vi "setBoundaries.vi"(8 "error in (no error)":errorcluster, 10 "Boundaries":T1, 11 "Rectangle in":refnum<class "Rectangle.lvclass">) -> (0 "error out":errorcluster, 3 "Rectangle out":refnum<class "Rectangle.lvclass">)   [LabVIEW 2010, in "Rectangle.lvclass"]
uses:
  Rectangle.lvclass
  Rectangle.lvclass/Rectangle.ctl
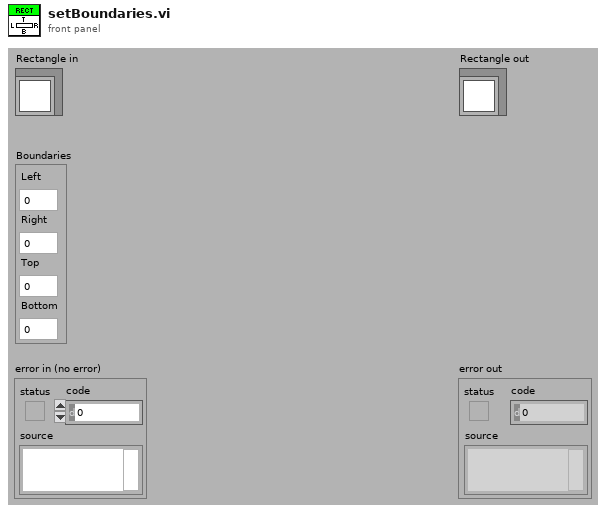
[diagram p1: front panel]
types:
  T1 = cluster{"Left":dbl, "Right":dbl, "Top":dbl, "Bottom":dbl}
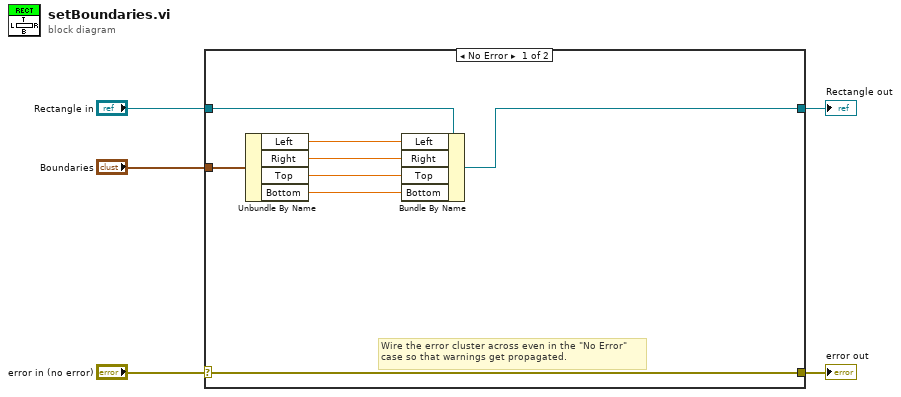
[diagram p0: block diagram]
diagram:
  n1 = case shown="No Error" "error in (no error)" {
    selector: "error in (no error)" -> [w13 w15]
    tunnel: [w13 w15] -> w4
    tunnel: [w11 w14] -> w2
    tunnel: "Rectangle in" -> [w12 w14]
    tunnel: "Boundaries" -> [w10 _]
    frame No Error {
      # "Wire the error cluster across even in the \"No Error\"\ncase so that warnings get propagated."
      n2 = Unbundle By Name(w10) -> ("Left"=w9:dbl, "Right"=w8:dbl, "Top"=w7:dbl, "Bottom"=w6:dbl)
      n3 = Bundle By Name(cluster=w12, "Left"=w9, "Right"=w8, "Top"=w7, "Bottom"=w6) -> (w11:refnum<class "Rectangle.lvclass">)
    }
    frame Error {
    }
  }
  "error out" <- w4
  "Rectangle out" <- w2
